vi "Apply Filters.vi"(8 "error in":errorcluster, 10 "Display State In":T1, 11 "MCListbox Refnum in":refnum<vi>) -> (0 "error out":errorcluster, 2 "Display State out":T1, 3 "MCListbox Refnum out":refnum<vi>)   [LabVIEW 2012, in "ListBox_XControl.xctl"]
doc: "Apply filters to the rows using the value filters in the X-control property.\nCan include lower limit and upper limit and column to apply. (applies filtering aphabetically)"
uses:
  ListBox_XControl.xctl
  ListBox_State.ctl
  Order Type Def.ctl
  Value Filters.ctl
  <userlib>/_OpenG.lib/array/array.llb/Delete Elements from 2D Array (String)__ogtk.vi
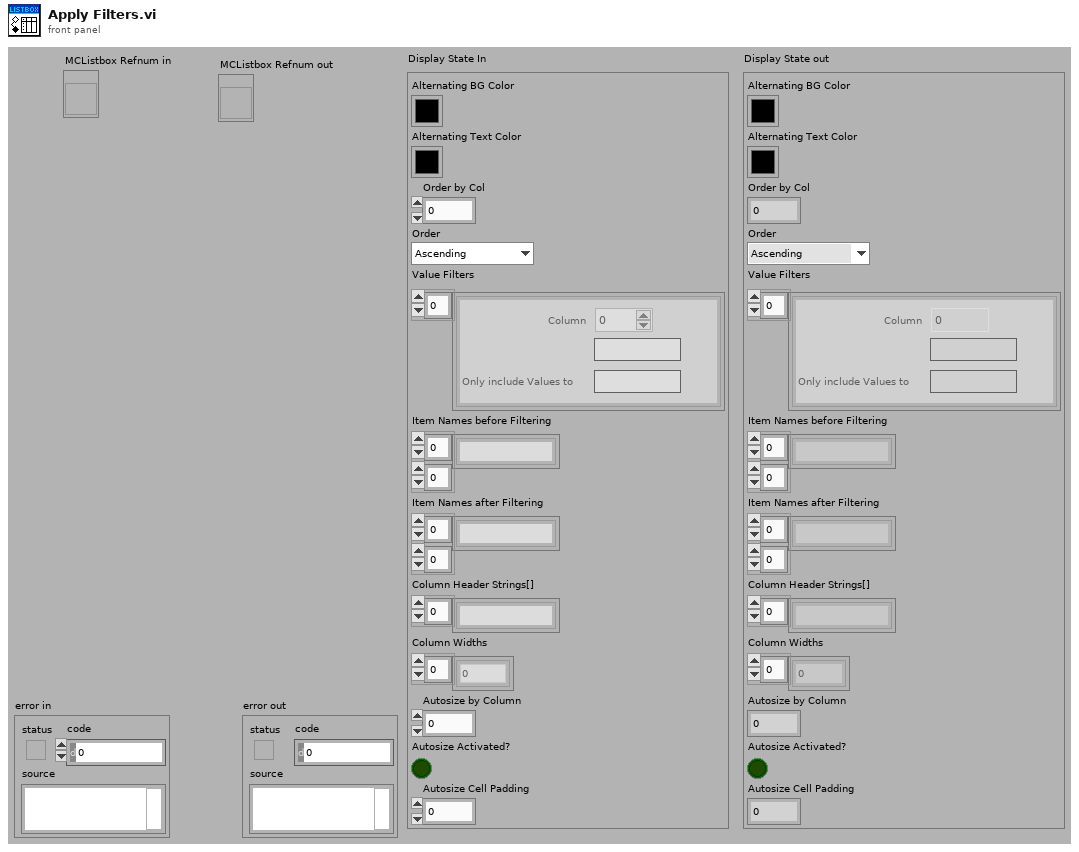
[diagram p1: front panel]
types:
  T1 = typedef "ListBox_XControl.xctl/ListBox_State.ctl" = cluster{"Alternating BG Color":u32, "Alternating Text Color":u32, "Order by Col":i32, "Order":T2, "Value Filters":T3, "Item Names before Filtering":string[][], "Item Names after Filtering":string[][], "Column Header Strings[]":string[], "Column Widths":u32[], "Autosize by Column":i32, "Autosize Activated?":bool, "Autosize Cell Padding":u32}
  T2 = typedef "ListBox_XControl.xctl/Order Type Def.ctl" = enum16{"Ascending", "Descending", "Off"}
  T3 = typedef "ListBox_XControl.xctl/Value Filters.ctl" = cluster{"Column":i32, "Only include Values From":string, "Only include Values to":string}[]
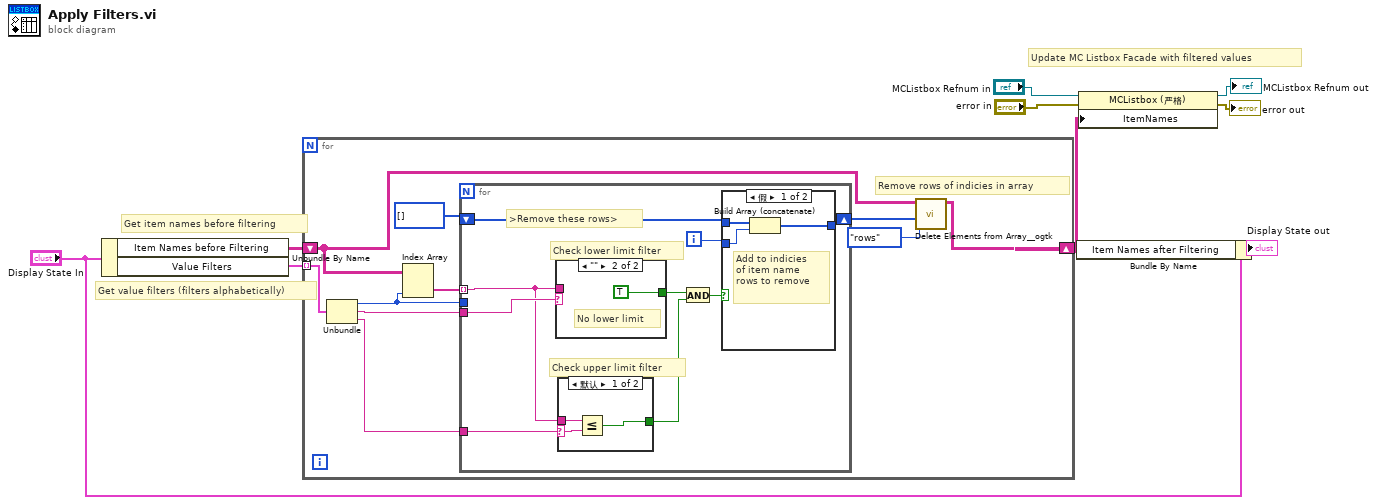
[diagram p0: block diagram]
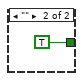
[diagram p2: hidden frame]
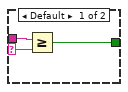
[diagram p3: hidden frame]
diagram:
  # "Update MC Listbox Facade with filtered values"
  # "Get value filters (filters alphabetically)"
  # "Get item names before filtering"
  n1 = Unbundle By Name("Display State In") -> ("Item Names before Filtering"=w4:string[][], "Value Filters"=w9:T3)
  n2 = for {
    tunnel: w9 -> [w19] mode=indexing
    shift-right: [w11] -> w2
    shift-left: w4 -> [w12]
    # "Remove rows of indicies in array"
    n3 = Unbundle(w19) -> ("Column"=w16:i32, "Only include Values From"=w18:string, "Only include Values to"=w17:string)
    n4 = Index Array(array=w12, index (col)=w16) -> (element=w15:string[])  [unwired: 1 in]
    n5 = for {
      shift-right: [w20] -> w13
      shift-left: i32[] [] -> [w23]
      tunnel: w18 -> [w28]
      tunnel: w17 -> [w27]
      tunnel: w16 -> [_]
      tunnel: w15 -> [w21] mode=indexing
      i -> [w22]
      # ">Remove these rows>"
      # "Check upper limit filter"
      # "Check lower limit filter"
      n6 = case shown="\"\"" w28 {
        selector: w28 -> [w35 _]
        tunnel: [w34 TRUE] -> w26
        tunnel: w21 -> [w33 _]
        frame Default {
          n7 = Greater Or Equal?(x=w33, y=w35) -> (x >= y?=w34:bool)
        }
        frame "" {
          # "No lower limit"
        }
      }
      n8 = case shown="默认" w27 {
        selector: w27 -> [w31 _]
        tunnel: [w30 TRUE] -> w24
        tunnel: w21 -> [w29 _]
        frame Default {
          n9 = Less Or Equal?(x=w29, y=w31) -> (x <= y?=w30:bool)
        }
        frame "" {
        }
      }
      n10 = And(x=w26, y=w24) -> (x .and. y?=w25:bool)
      n11 = case shown="假" w25 {
        tunnel: w23 -> [w39 w40]
        tunnel: w22 -> [w38 _]
        tunnel: [w37 w40] -> w20
        frame False {
          # "Add to indicies\nof item name\nrows to remove"
          n12 = Build Array (concatenate)(w39, w38) -> (w37:i32[])
        }
        frame True {
        }
      }
    }
    n13 = call-poly <userlib>:"Delete Elements from Array__ogtk.vi"("delete (rows or columns)"=enum16{"rows", "columns"}."rows", "indices"=w13, "array"=w12) -> ("array w/ subset deleted"=w11:string[][])  [unwired: 7 in, 1 out]
  }
  n14 = Bundle By Name(cluster="Display State In", "Item Names after Filtering"=w2) -> (→"Display State out":T1)
  n15 = property class="MCListbox (严格)"(reference="MCListbox Refnum in", error in="error in", "ItemNames"=w2) -> (reference out=→"MCListbox Refnum out":refnum<vi>, error out=→"error out":errorcluster)
